vi "WPI_DashboardSave DB Images.vi"(5 "Path":path, 6 "Images to Keep":dbl=180.0, 7 "Time Interval (s)":dbl=1.0, 8 "Camera Name":string="Camera ", 9 "Image":T1) -> ()   [LabVIEW 2017]
doc: "This VI saves the most recent images at a specified interval. It saves them to the provided path or to the public documents/FRC/DV Images directory. The name is composed of the camera name and the image sequence number."
uses:
  <vilib>/Utility/sysdir.llb/System Directory Type.ctl
  <vilib>/vision/Image Controls.llb/IMAQ Image.ctl
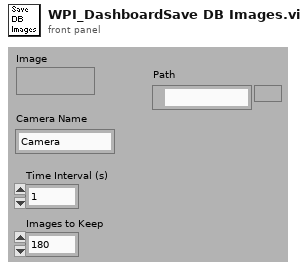
[diagram p1: front panel]
types:
  T1 = typedef "IMAQ Image.ctl" = refnum<image>
  T2 = typedef "System Directory Type.ctl" = i32
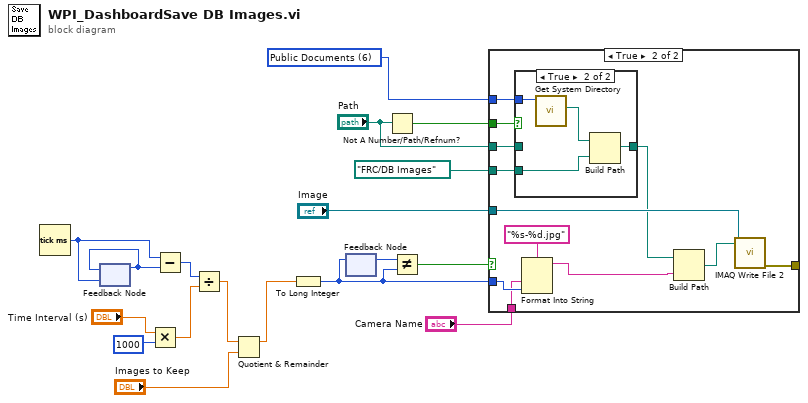
[diagram p0: block diagram]
diagram:
  w3 = T2 6 items=["User Home"=0, "User Desktop"=1, "User Documents"=2, "User Application Data"=3, "User Preferences"=4, "User Temporary"=5, "Public Documents"=6, "Public Application Data"=7, "Public Preferences"=8, "Public Cache"=13, "System Core Libraries"=9, "System Installed Libraries"=10, "Application Files"=11, "Boot Volume Root"=12] ("system directory type")
  n1 = Tick Count (ms)() -> (millisecond timer value=w14:u32)
  n2 = feedback #1(w14) -> (w13:u32)
  n3 = feedback-in #1(w13) -> ()
  n4 = Multiply(x="Time Interval (s)", y=1000) -> (x*y=w10:dbl)
  n5 = Subtract(x=w14, y=w13) -> (x-y=w16:u32)
  n6 = Divide(x=w16, y=w10) -> (x/y=w7:dbl)
  n7 = Quotient & Remainder(x=w7, y="Images to Keep") -> (x-y*floor(x/y)=w6:dbl)  [unwired: 1 out]
  n8 = To Long Integer(number=w6) -> (32bit integer=w8:i32)
  n9 = feedback-in #2(w8) -> ()
  n10 = feedback #2() -> (w17:i32)  [unwired: 1 out]
  n11 = Not A Number/Path/Refnum?(number/path/refnum="Path") -> (NaN/Path/Refnum?=w5:bool)
  n12 = Not Equal?(x=w17, y=w8) -> (x != y?=w18:bool)
  n13 = case shown="True" w18 {
    tunnel: "Image" -> [_ w30]
    tunnel: [_ w28] -> _
    tunnel: w8 -> [_ w20]
    tunnel: w5 -> [_ w26]
    tunnel: "Path" -> [_ w25]
    tunnel: path "FRC/DB Images" -> [_ w23]
    tunnel: w3 -> [_ w22]
    tunnel: "Camera Name" -> [_ w19]
    frame False {
    }
    frame True {
      n14 = case shown="True" w26 {
        tunnel: w25 -> [w31 _]
        tunnel: [w31 w35] -> w24
        tunnel: w23 -> [_ w34]
        tunnel: w22 -> [_ w33]
        frame False {
        }
        frame True {
          n15 = call <vilib>:"Get System Directory.vi"("system directory type"=w33) -> ("system directory"=w32:path)  [unwired: 10 in]
          n16 = Build Path(base path=w32, name or relative path=w34) -> (appended path=w35:path)
        }
      }
      n17 = Format Into String(format string="%s-%d.jpg", w19, w20) -> (resulting string=w27:string)  [unwired: 2 in, 1 out]
      n18 = Build Path(base path=w24, name or relative path=w27) -> (appended path=w29:path)
      n19 = call-poly "IMAQ Write File 2"("File Path"=w29, "Image"=w30) -> ("error out"=w28:errorcluster)  [unwired: 3 in, 6 out]
    }
  }
